vi "Periodic Tasks.vi"(8 "error in":errorcluster) -> ()   [LabVIEW 2023]
doc: "This VI runs in parallel to other robot code. It can contain as many user-defined periodic loops as you need. These can carry out PID or other sorts of timed response."
uses:
  bordeaux-pathinator/Bordeaux/Types/Segment Type.ctl
  <vilib>/Analysis/coordinate.llb/Angle Units.ctl
  bordeaux-pathinator/Bordeaux/Types/Angluar Limits.ctl
  bordeaux-pathinator/Bordeaux/Types/Limits.ctl
  <vilib>/Analysis/coordinate.llb/Wrap Angle (scalar).vi
  <vilib>/Rock Robotics/WPI/ThirdParty/Phoenix-LabVIEW/Pigeon IMU/CTRE_PigeonIMU_GetYPR.vi
  <vilib>/Rock Robotics/Network Tables/NT Write Number.vi
  <vilib>/Analysis/NI_AAL_Angle.lvlib
panel:
  in  "WayPoints":cluster{"x":dbl, "y":dbl, "th":dbl}[](array[cluster])
  out "Trajectory Data Out":T2(array[cluster])
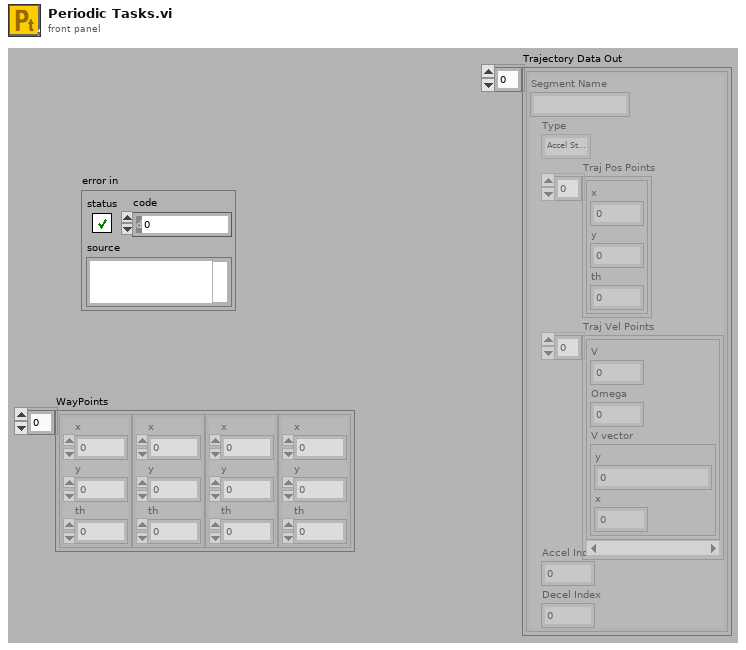
[diagram p1: front panel]
types:
  T1 = typedef "Segment Type.ctl" = enum16{"Accel Straight", "Const Straight", "Blend", "Circle", "Bezier"}
  T2 = cluster{"Segment Name":string, "Type":T1, "Traj Pos Points":cluster{"x":dbl, "y":dbl, "th":dbl}[], "Traj Vel Points":cluster{"V":dbl, "Omega":dbl, "V vector":cluster{"y":dbl, "x":dbl}}[], "Accel Index":i32, "Decel Index":i32}[]
  T3 = typedef "Limits.ctl" = cluster{"Velocity (fps)":dbl, "Accel (fps^2)":dbl, "Jerk (fps^3)":dbl, "StoopidFast (fps)":dbl}
  T4 = typedef "Angluar Limits.ctl" = cluster{"Velocity (deg/s)":dbl, "Accel (deg/s^2)":dbl, "Jerk (deg/s^3)":dbl}
  T5 = typedef "NI_AAL_Angle.lvlib/Angle Units.ctl" = i32
  T6 = typedef "CTRE_PigeonIMU_DeviceRef.ctl" = cluster{"DeviceStatus":errorcluster, "Device Number":u8, "Type":T7, "Device ID":u32, "Handle":u64, "UsageFrame":u32, "Library Path":path}
  T7 = typedef "CTRE_PigeonIMU_ConnectionType.ctl" = u32
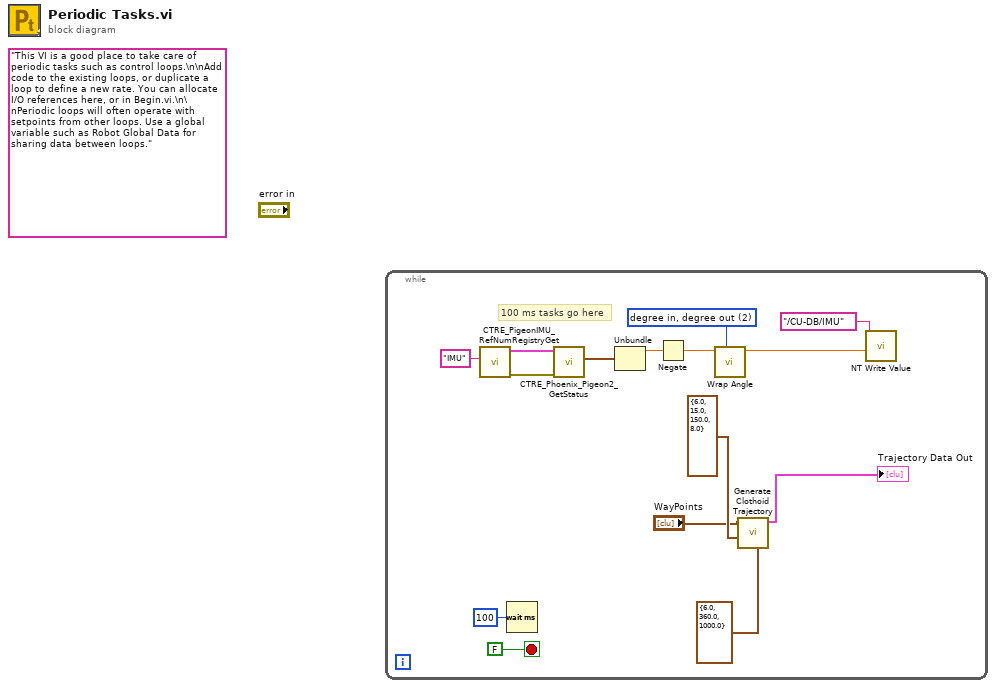
[diagram p0: block diagram]
diagram:
  (unwired) "This VI is a good place to take care of periodic tasks such as control loops.\n\nAdd code to the existing loops, or duplicate a loop to define a new rate. You can allocate I/O references here, or in Begin.vi.\n\nPeriodic loops will often operate with setpoints from other loops. Use a global variable such as Robot Global Data for sharing data between loops."
  n1 = while {
    stop <- FALSE stop-if-true
    w5 = T5 2 items=["radian in, radian out", "radian in, degree out", "degree in, degree out", "degree in, radian out"] ("angle units")
    # "100 ms tasks go here"
    n2 = call <vilib>:"CTRE_PigeonIMU_RefNumRegistryGet.vi"("refnum name"="IMU") -> ("error out"=w12:errorcluster, "PigeonIMUDevRef"=w11:T6)  [unwired: 9 in]
    n3 = Wait (ms)(milliseconds to wait=u32 100) -> ()  [unwired: 1 out]
    n4 = call-poly <vilib>:"CTRE_Phoenix_Pigeon2_GetStatus.vi"("error in (no error)"=w12, "PigeonIMUDevRef"=w11) -> ("Yaw Pitch Roll"=w13:cluster{"Yaw":dbl, "Pitch":dbl, "Roll":dbl})  [unwired: 7 in, 2 out]
    n5 = Unbundle(w13) -> ("Yaw"=w8:dbl)  [unwired: 2 out]
    n6 = Negate(x=w8) -> (-x=w7:dbl)
    n7 = call-poly <vilib>:"Wrap Angle.vi"("angle units"=w5, "angle in"=w7) -> ("angle out"=w6:dbl)  [unwired: 8 in, 1 out]
    n8 = call "Generate Clothoid Trajectory.vi"("Angular Limits"=T4 {"Velocity (deg/s)"=6.0, "Accel (deg/s^2)"=360.0, "Jerk (deg/s^3)"=1000.0}, "Limits"=T3 {"Velocity (fps)"=6.0, "Accel (fps^2)"=15.0, "Jerk (fps^3)"=150.0, "StoopidFast (fps)"=8.0}, "WayPoints"="WayPoints") -> ("Trajectory Data Out"=→"Trajectory Data Out":T2)  [unwired: 5 in, 3 out]
    n9 = call-poly <vilib>:"NT Write Value.vi"("value"=w6, "name"="/CU-DB/IMU") -> ()  [unwired: 9 in, 1 out]
  }
